vi "Tree_DragDrop_Event Handler.vi"(11 "Tree Ref Array":refnum<vi>[](array[refnum])) -> ()   [LabVIEW 2023]
doc: "Sync multiple trees. Drag and drop within one tree will be repeated for the other trees. Currently does not work for dropping on item (indenting). can only work reliably on non-indented flat trees).\n\nWhen drag is over, deselect items."
panel:
  in  "Tree 3":string(tree)
  in  "Tree 2":string(tree)
  in  "Items Ct":i32
  in  "Tree 1":string[](tree)
  # "we're going to have to set up a user event for other changes, such as programatic open and close due to filtering. UE for top item changed"
  # "For debug"
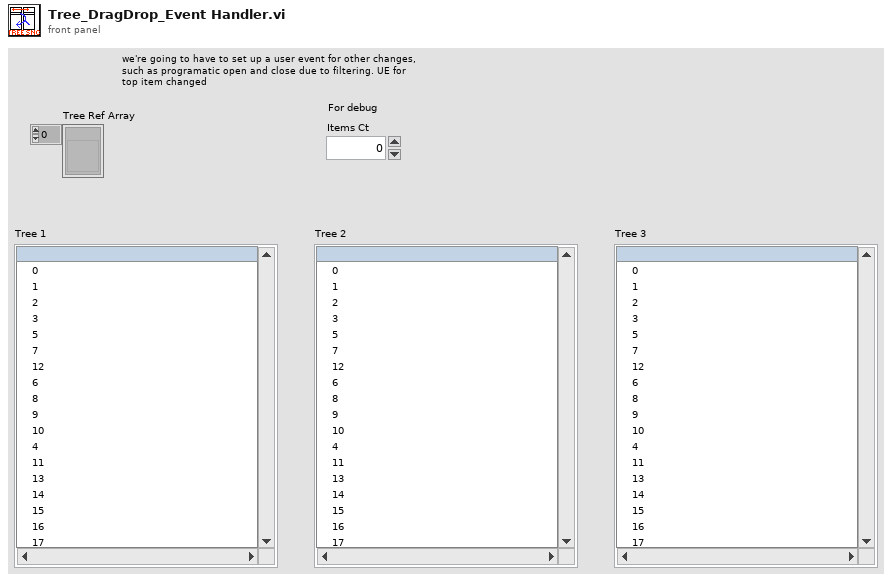
[diagram p1: front panel]
types:
  T1 = cluster{"Start index":i32, "Start Tag":string, "Value on Drag":string[]}
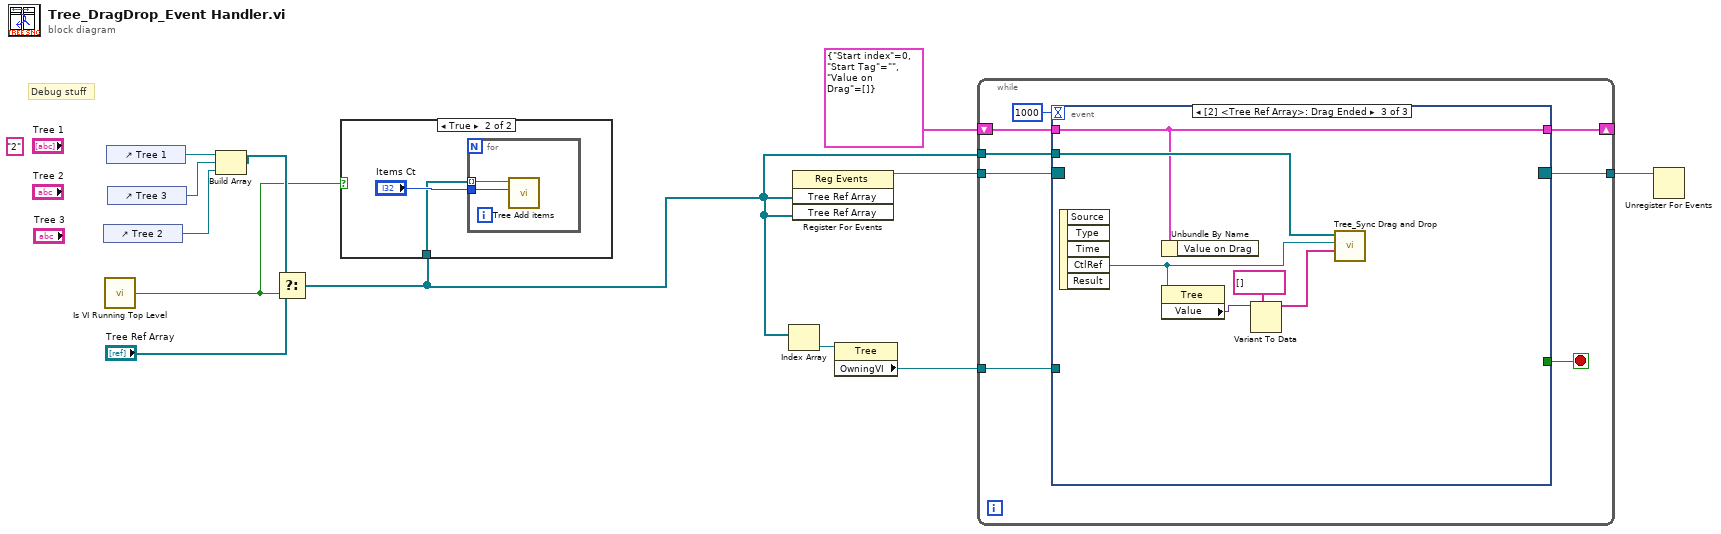
[diagram p0: block diagram]
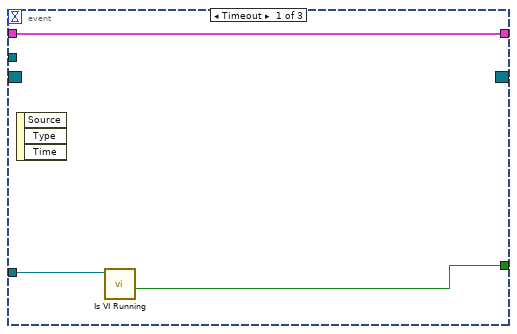
[diagram p3: hidden frame]
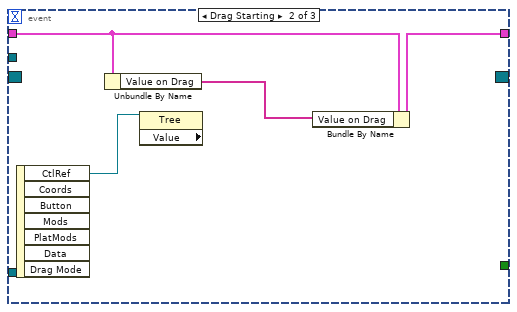
[diagram p4: hidden frame]
diagram:
  (unwired) "2" ("Tree 1")
  # "Debug stuff"
  n1 = control-ref of="Tree 2"() -> (w9:refnum<vi>)
  n2 = call "Is VI Running Top Level.vi"() -> ("Top Level?"=w6:bool)  [unwired: 5 in]
  n3 = control-ref of="Tree 1"() -> (w12:refnum<vi>)
  n4 = control-ref of="Tree 3"() -> (w11:refnum<vi>)
  n5 = Build Array(w12, w11, w9) -> (w7:refnum<vi>[])
  n6 = Select(t=w7, s=w6, f="Tree Ref Array") -> (s? t:f=w3:refnum<vi>[])
  n7 = case shown="True" w6 {
    tunnel: w3 -> [_ w13]
    frame False {
    }
    frame True {
      n8 = for {
        tunnel: "Items Ct" -> [w16]
        tunnel: w13 -> [w15] mode=indexing
        n9 = call "Tree Add items.vi"("Items Ct"=w16, "TreeControl in"=w15) -> ()  [unwired: 9 in, 1 out]
      }
    }
  }
  n10 = Index Array(array=w3) -> (element=w5:refnum<vi>)  [unwired: 1 in]
  n11 = register-events(w3, w3) -> (reference out=w10:refnum<event-registration>)  [unwired: 2 in, 1 out]
  n12 = property class="Tree"(reference=w5) -> ("OwningVI"=w4:refnum<vi>)  [unwired: 1 in, 2 out]
  n13 = while {
    tunnel: w10 -> [w23]
    tunnel: w3 -> [w22]
    tunnel: w4 -> [w21]
    tunnel: [w19] -> w2
    shift-right: [w18] -> _
    shift-left: T1 {"Start index"=0, "Start Tag"="", "Value on Drag"=[]} -> [w17]
    stop <- w24 stop-if-true
    n14 = event shown="[2] <Tree Ref Array>: Drag Ended" {
      selector: w23 -> [_ _ _]
      dyn-events: [_ _ _] -> w19
      timeout: 1000 -> [_ _ _]
      tunnel: [w26 _ _] -> w24
      tunnel: w22 -> [_ _ w37]
      tunnel: w21 -> [w27 _ _]
      tunnel: [w25 w31 w36] -> w18
      tunnel: w17 -> [w25 w29 w36]
      event Timeout {
        n15 = event-data() -> ()  [unwired: 1 in, 3 out]
        n16 = call "Is VI Running.vi"("VI in"=w27) -> ("VI Not Running"=w26:bool)  [unwired: 7 in, 3 out]
      }
      event Drag Starting {
        n17 = event-data() -> ("CtlRef"=w30:refnum<vi>)  [unwired: 1 in, 6 out]
        n18 = Unbundle By Name(w29) -> ("Value on Drag"=w28:string[])
        n19 = property class="Tree" props=["Value"](reference=w30) -> ()  [unwired: 1 in, 3 out]
        n20 = Bundle By Name(cluster=w29, "Value on Drag"=w28) -> (w31:T1)
      }
      event Drag Ended {
        n21 = event-data() -> ("CtlRef"=w35:refnum<vi>)  [unwired: 1 in, 4 out]
        n22 = Unbundle By Name(w36) -> ()  [unwired: 1 out]
        n23 = property class="Tree"(reference=w35) -> ("Value"=w34:variant)  [unwired: 1 in, 2 out]
        n24 = Variant To Data(type=string[] [] ("Value on Drag"), Variant=w34) -> (data=w32:string[])  [unwired: 1 in, 1 out]
        n25 = call "Tree_Sync Drag and Drop.vi"("Value on Drag"=w32, "TreeControl in"=w35, "Tree Ref Array"=w37) -> ()  [unwired: 9 in]
      }
    }
  }
  n26 = Unregister For Events(event registration refnum=w2) -> ()  [unwired: 1 in, 1 out]
